vi "ActorDatabase-PerformUpdate.vi"(8 "error in (no error)":errorcluster, 11 "Database-Actor in":refnum<class "Database-Actor.lvclass">) -> (0 "error out":errorcluster, 2 "Update Successful":bool, 3 "Database-Actor out":refnum<class "Database-Actor.lvclass">)   [LabVIEW 2013, in "Database-Actor.lvclass"]
uses:
  Database-Actor.lvclass
  Database-Actor.lvclass/Database-Actor.ctl
  ftw-dataflow/Core/src/JSON/FTW-JSON-RegexParse.vi
  ftw-dataflow/Core/src/Error/FTW-ERR-ThrowGenericError.vi
  ftw-dataflow/Core/src/Container/FTW-Container-Construct.vi
  ftw-dataflow/Core/src/Container/FTW-Container-Load-JSON.vi
  ftw-dataflow/Core/src/Container/FTW-Container-Destroy.vi
  ftw-dataflow/Core/utils/CodeGen/JSON Deserialize/FTW-JSON-Deserialize.xnode
  Reuse Library/Database API/Database-API.lvclass
  ftw-dataflow/Core/src/Container/FTW-Container.lvclass
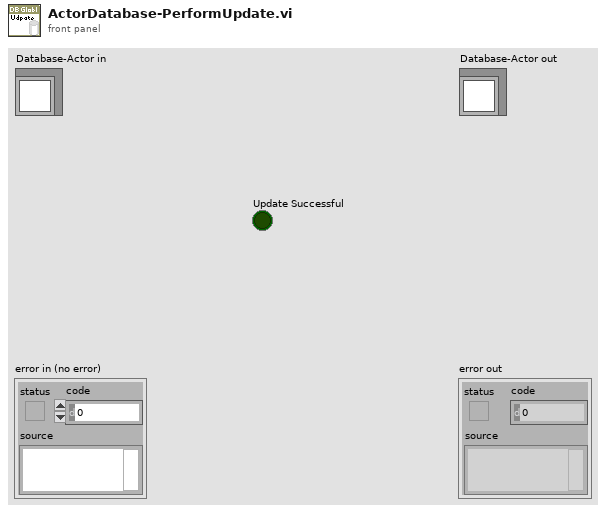
[diagram p1: front panel]
types:
  T1 = cluster{"Table":string, "SQL Statement":string, "Update All":bool, "Payload":string, "Column Number":i32, "Datatype":i32}
  T2 = cluster{"Path for Picture Material":path, "Path for Picture Material 2":path, "Path for Picture Material 3":path, "Path for Picture Material 4":path, "Path for Picture Material 5":path, "Path for Picture Material 6":path, "Path for Picture Material 7":path, "Get Material Instruction":string}[]
  T3 = cluster{"[0]":string, "[1]":string, "[2]":string, "[3]":string, "[4]":string, "[5]":string, "[6]":string, "[7]":string, "[8]":string}
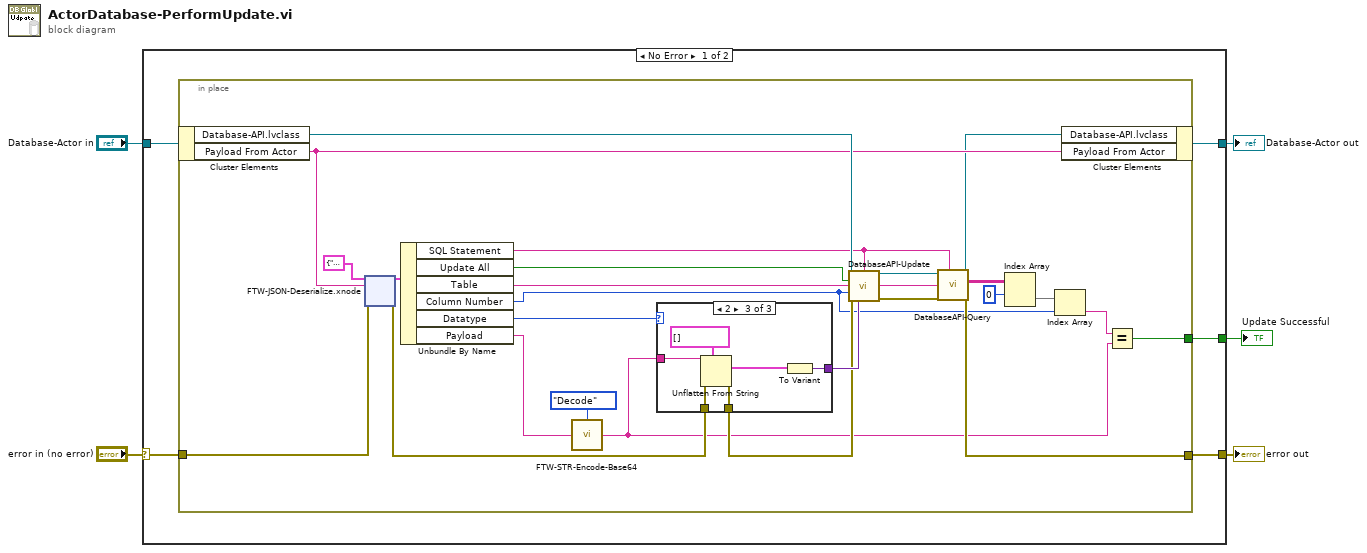
[diagram p0: block diagram]
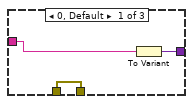
[diagram p2: hidden frame]
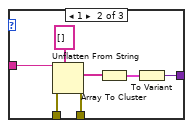
[diagram p3: hidden frame]
diagram:
  n1 = case shown="No Error" "error in (no error)" {
    selector: "error in (no error)" -> [w8 w86]
    tunnel: [w7 w86] -> w4
    tunnel: [w9 w85] -> w2
    tunnel: "Database-Actor in" -> [w10 w85]
    tunnel: [w6 _] -> w1
    frame No Error {
      n2 = in-place {
        in-place-border: w8 -> [w33]
        in-place-border: [w23] -> w7
        in-place-border: [w11] -> w6
        n3 = in-place-cluster #1(w10) -> ("Database-API.lvclass"=w35:refnum<class "Database-API.lvclass">, "Payload From Actor"=w32:string)
        n4 = xnode "FTW-JSON-Deserialize.xnode"("Data Type and Default Values"=T1 {"Table"="", "SQL Statement"="", "Update All"=FALSE, "Payload"="", "Column Number"=0, "Datatype"=0} ("output cluster"), "JSON String"=w32, "error in"=w33) -> ("Populated Values"=w34:T1, "error out"=w19:errorcluster)
        n5 = Unbundle By Name(w34) -> ("SQL Statement"=w27:string, "Update All"=w31:bool, "Table"=w25:string, "Column Number"=w14:i32, "Datatype"=w21:i32, "Payload"=w20:string)
        n6 = call "FTW-STR-Encode-Base64.vi"("Input"=w20, "Direction"=enum16{"Encode", "Decode"}."Decode") -> ("Output"=w12:string)
        n7 = case shown="2" w21 {
          tunnel: w12 -> [w37 w44 w51]
          tunnel: [w38 w41 w50] -> w28
          tunnel: w19 -> [w36 w40 w49]
          tunnel: [w36 w39 w48] -> w18
          frame 0, Default {
            n8 = To Variant(anything=w37) -> (Variant=w38:variant)
          }
          frame 1 {
            n9 = Unflatten From String(type=string[] [], binary string=w44, error in (no error)=w40) -> (value=w43:string[], error out=w39:errorcluster)  [unwired: 2 in, 1 out]
            n10 = Array To Cluster(array=w43) -> (cluster=w42:T3)
            n11 = To Variant(anything=w42) -> (Variant=w41:variant)
          }
          frame 2 {
            n12 = Unflatten From String(type=T2 [] ("appended array"), binary string=w51, error in (no error)=w49) -> (value=w46:T2, error out=w48:errorcluster)  [unwired: 2 in, 1 out]
            n13 = To Variant(anything=w46) -> (Variant=w50:variant)
          }
        }
        n14 = call "DatabaseAPI-Update.vi"("Database-API in"=w35, "data"=w28, "Where Statement"=w27, "Update All"=w31, "Table"=w25, "Column Number"=w14, "error in (no error)"=w18) -> ("Database-API out"=w26:refnum<class "Database-API.lvclass">, "error out"=w24:errorcluster)  [unwired: 7 in]
        n15 = call "DatabaseAPI-Query.vi"("optional clause"=w27, "error in (no error)"=w24, "Table"=w25, "Database-API in"=w26) -> ("error out"=w23:errorcluster, "data"=w17:string[][], "Database-API out"=w22:refnum<class "Database-API.lvclass">)  [unwired: 4 in, 1 out]
        n16 = Index Array(array=w17, index (row)=0) -> (element=w15:string[])  [unwired: 1 in]
        n17 = Index Array(array=w15, index=w14) -> (element=w13:string)
        n18 = in-place-cluster #1("Database-API.lvclass"=w22, "Payload From Actor"=w32) -> (w9:refnum<class "Database-Actor.lvclass">)
        n19 = Equal?(x=w13, y=w12) -> (x = y?=w11:bool)
      }
    }
    frame Error {
    }
  }
  "error out" <- w4
  "Database-Actor out" <- w2
  "Update Successful" <- w1
